vi "runServer.vi"(8 "error in (no error)":errorcluster, 11 "TcpServerBase in":refnum<class "TcpServerBase.lvclass">) -> (0 "error out (no error)":errorcluster, 3 "TcpServerBase out":refnum<class "TcpServerBase.lvclass">)   [LabVIEW 2018, in "TcpServerBase.lvclass"]
doc: "Run the TCP Server Base.\n\nNOTE: Server Queue and Client Queue are destroyed in \"stop server\" state inside of tcpServerStateMachine.vi"
uses:
  TcpServerBase.lvclass
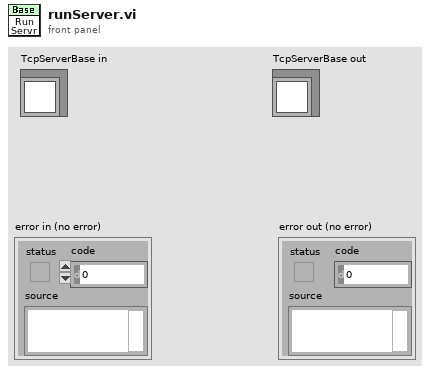
[diagram p1: front panel]
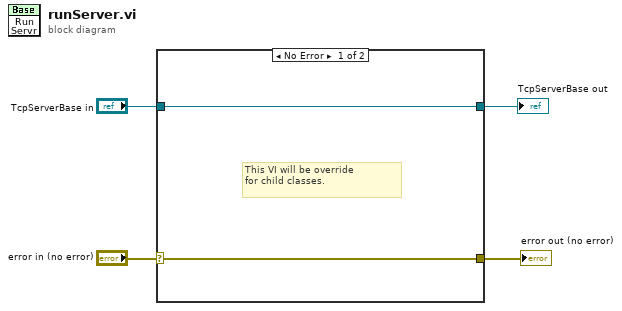
[diagram p0: block diagram]
diagram:
  n1 = case shown="No Error" "error in (no error)" {
    selector: "error in (no error)" -> [w6 w7]
    tunnel: [w6 w7] -> w3
    tunnel: [w5 w8] -> w2
    tunnel: "TcpServerBase in" -> [w5 w8]
    frame No Error {
      # "This VI will be override\nfor child classes."
    }
    frame Error {
    }
  }
  "error out (no error)" <- w3
  "TcpServerBase out" <- w2
